vi "solar_tcp Identify.vi"(10 "TCP Data":T1={"Connected"=FALSE, "Config"={"TCPServer"=enum."SERVER", "ServerPort"=0, "IPAddress"="", "ClientPort"=0, "HdrSizeBytes"=4, "HdrLenSubtractBytes"=0, "HdrLenOffsetBits"=0, "HdrLenSizeBits"=32}, "Clients"=[], "ConnectionID"=refnum, "Debug"=[]} {"Debug"."Time" format="%<%Y-%m-%d\n%H:%M:%S%3u>T"}) -> (1 "Connected?":bool, 2 "Identify":string, 4 "Valid ConnectionID?":bool, 5 "TCPServer":enum8{"SERVER", "CLIENT"}(ring))   [LabVIEW 2018]
doc: "This returns a unique TCP connection identifier:\nTCP Server: '<name>(<server_port>)'\nTCP Client: '<name>(<client_port>-<server_ip>:<server_port>)'\n\nExamples:\nMyServer(59300)\nMyClient(59300-localhost:59200)"
uses:
  solar_tcp_ctl Data.ctl
  solar_tcp_ctl Config.ctl
  solar_tcp_ctl Action.ctl
  solar_tcp_ctl Debug.ctl
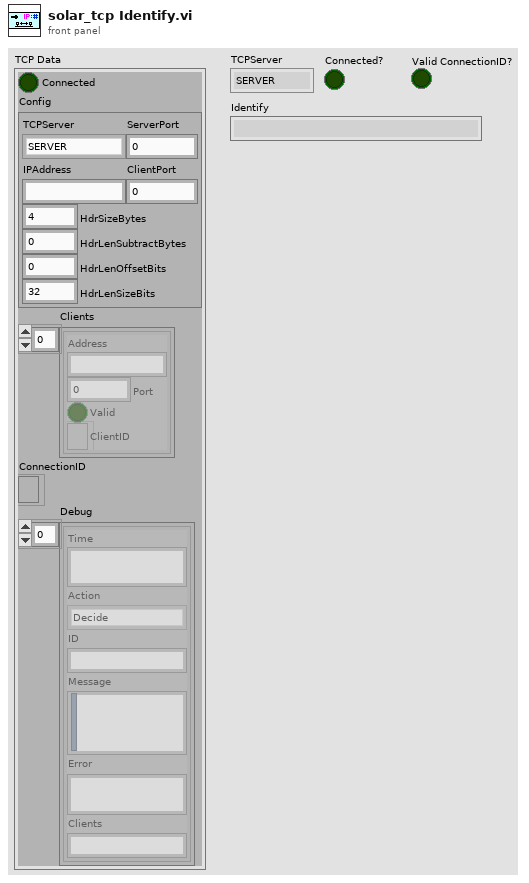
[diagram p1: front panel]
types:
  T1 = typedef "solar_tcp_ctl Data.ctl" = cluster{"Connected":bool, "Config":T2, "Clients":cluster{"Address":string, "Port":u16, "Valid":bool, "ClientID":refnum<k5>}[], "ConnectionID":refnum<k5>, "Debug":T3[]}
  T2 = typedef "solar_tcp_ctl Config.ctl" = cluster{"TCPServer":enum8{"SERVER", "CLIENT"}, "ServerPort":u16, "IPAddress":string, "ClientPort":u16, "HdrSizeBytes":i32, "HdrLenSubtractBytes":i32, "HdrLenOffsetBits":i32, "HdrLenSizeBits":i32}
  T3 = typedef "solar_tcp_ctl Debug.ctl" = cluster{"Time":timestamp, "Action":T4, "ID":string, "Message":string, "Error":string, "Clients":string}
  T4 = typedef "solar_tcp_ctl Action.ctl" = enum16{"Decide", "CreateListener", "Open", "Read", "Write", "Close", "Shutdown", "Done", "ChangePort"}
  T5 = cluster{"Address":string, "Port":u16, "Valid":bool, "ClientID":refnum<k5>}[]
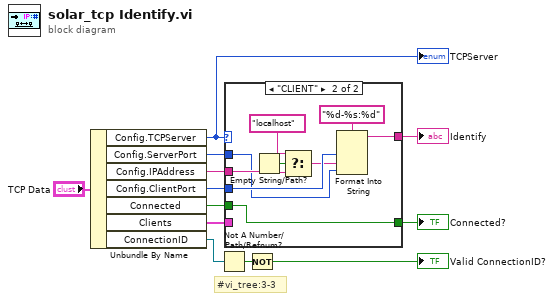
[diagram p0: block diagram]
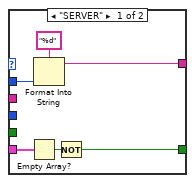
[diagram p2: hidden frame]
diagram:
  # "#vi_tree:3-3"
  n1 = Unbundle By Name("TCP Data") -> ("Config.TCPServer"=w11:enum8{"SERVER", "CLIENT"}, "Config.ServerPort"=w10:u16, "Config.IPAddress"=w9:string, "Config.ClientPort"=w8:u16, "Connected"=w5:bool, "Clients"=w7:T5, "ConnectionID"=w3:refnum<k5>)
  "TCPServer" <- w11
  n2 = Not A Number/Path/Refnum?(number/path/refnum=w3) -> (NaN/Path/Refnum?=w2:bool)
  n3 = case shown="\"CLIENT\"" w11 {
    tunnel: w10 -> [w18 w19]
    tunnel: w9 -> [_ w22]
    tunnel: w8 -> [_ w27]
    tunnel: [w17 w26] -> w4
    tunnel: w7 -> [w16 _]
    tunnel: [w14 w25] -> w6
    tunnel: w5 -> [_ w25]
    frame "SERVER" {
      n4 = Empty Array?(array=w16) -> (empty?=w15:bool)
      n5 = Format Into String(format string="%d", w18) -> (resulting string=w17:string)  [unwired: 2 in, 1 out]
      n6 = Not(x=w15) -> (.not. x?=w14:bool)
    }
    frame "CLIENT" {
      n7 = Empty String/Path?(string/path=w22) -> (empty?=w24:bool)
      n8 = Select(t="localhost", s=w24, f=w22) -> (s? t:f=w21:string)
      n9 = Format Into String(format string="%d-%s:%d", w27, w21, w19) -> (resulting string=w26:string)  [unwired: 2 in, 1 out]
    }
  }
  "Identify" <- w4
  "Connected?" <- w6
  n10 = Not(x=w2) -> (.not. x?=→"Valid ConnectionID?":bool)
